vi "InitTasks_PXI.vi"() -> (3 "PXI_Cluster":T1[](array[typedef]))   [LabVIEW 2013]
uses:
  AcqControls/Tasks_Indices.ctl
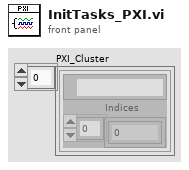
[diagram p1: front panel]
types:
  T1 = typedef "Tasks_Indices.ctl" = cluster{"task out":refnum<k21>, "Indices":i32[]}
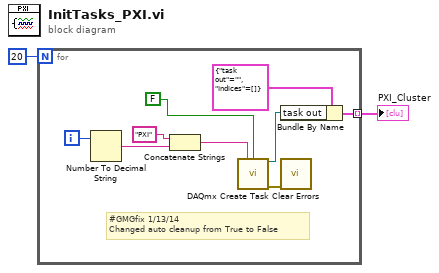
[diagram p0: block diagram]
diagram:
  n1 = for {
    N: 20 -> [_]
    tunnel: [w4] -> w2 mode=indexing
    i -> [w8]
    # "#GMGfix 1/13/14 \nChanged auto cleanup from True to False"
    n2 = Number To Decimal String(number=w8) -> (decimal integer string=w10:string)  [unwired: 1 in]
    n3 = Concatenate Strings("PXI" ("string"), w10) -> (w9:string)
    n4 = call <vilib>:"DAQmx Create Task.vi"("new task name"=w9, "auto cleanup"=FALSE) -> ("task out"=w5:refnum<k21>, "error out"=w7:errorcluster)  [unwired: 3 in, 9 out]
    n5 = Bundle By Name(cluster=T1 {"task out"="", "Indices"=[]} ("Tasks+Indices"), "task out"=w5) -> (w4:T1)
    n6 = call <vilib>:"Clear Errors.vi"("error in (no error)"=w7) -> ()  [unwired: 6 in, 1 out]
  }
  "PXI_Cluster" <- w2
